vi "UDP_Send&Receive.vi"(4 "connection ID":refnum<k16>, 5 "In":string, 6 "timeout ms (2000)":i32=2000, 7 "error in (no error)":errorcluster, 8 "Read (TRUE)":bool, 9 "Address":u32=64 format="%.0x", 10 "IP address":string="192.168.10.20") -> (0 "error out":errorcluster={"status"=TRUE, "code"=56, "source"="UDP Read in UDP.vi->flash.vi"}, 1 "Out":u8 format="%.0x", 2 "received string":string, 3 "connection ID out":refnum<k16>)   [LabVIEW 2017]
panel:
  out "字符串":string
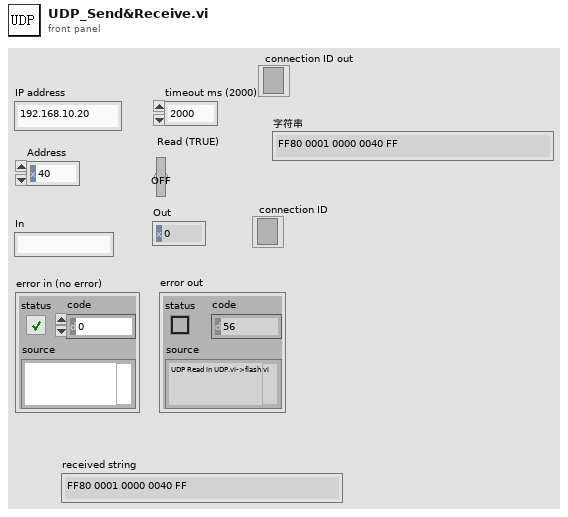
[diagram p1: front panel]
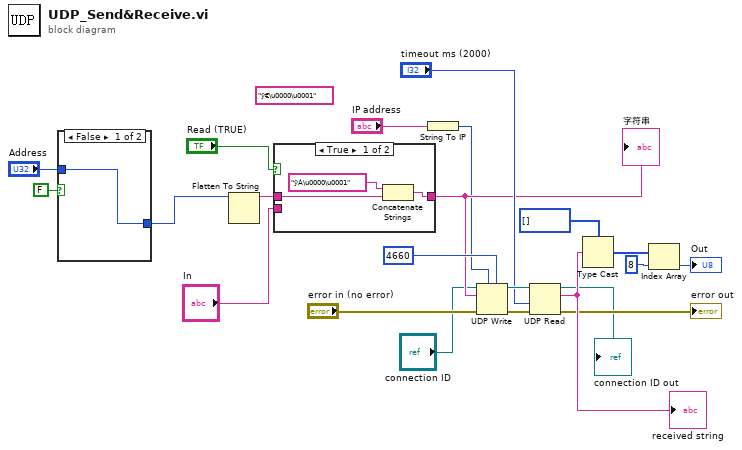
[diagram p0: block diagram]
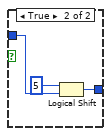
[diagram p2: hidden frame]
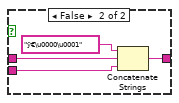
[diagram p3: hidden frame]
diagram:
  (unwired) "ÿ€\u0000\u0001" ("initial string")
  n1 = case shown="False" FALSE {
    tunnel: [w23 w25] -> w9
    tunnel: "Address" -> [w23 w24]
    frame False {
    }
    frame True {
      n2 = Logical Shift(y=i16 5, x=w24) -> (x << y=w25:u32)
    }
  }
  n3 = Flatten To String(anything=w9) -> (data string=w16:string)  [unwired: 3 in, 2 out]
  n4 = case shown="True" "Read (TRUE)" {
    tunnel: [w28 w32] -> w17
    tunnel: w16 -> [w27 w31]
    tunnel: "In" -> [_ w30]
    frame True {
      n5 = Concatenate Strings("ÿÀ\u0000\u0001" ("initial string"), w27) -> (w28:string)
    }
    frame False {
      n6 = Concatenate Strings("ÿ€\u0000\u0001" ("initial string"), w31, w30) -> (w32:string)
    }
  }
  "字符串" <- w17
  n7 = String To IP(1:"IP address") -> (0:w10:u32)
  n8 = UDP Write(address=w10, port or service name=u16 4660 ("UDP port"), connection ID="connection ID", data in=w17, 8:"error in (no error)") -> (error out=w19:errorcluster, 3:w20:refnum<k16>)  [unwired: 1 in]
  n9 = UDP Read(connection ID=w20, timeout ms (25000)="timeout ms (2000)", 8:w19) -> (data out=w6:string, error out=→"error out":errorcluster, 3:→"connection ID out":refnum<k16>)  [unwired: 3 out]
  "received string" <- w6
  n10 = Type Cast(type=u8[] [], x=w6) -> (*(type *) &x=w13:u8[])
  n11 = Index Array(array=w13, index=8) -> (element=→"Out":u8)
